vi "ConvStringIntoDouble (SubVI).vi"(1 "String In":string) -> (0 "Array Out":dbl[](array[numeric]))   [LabVIEW 2018]
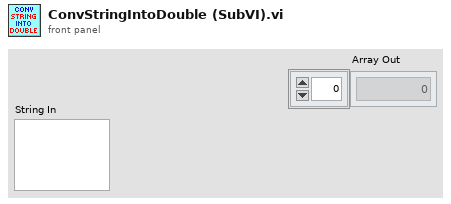
[diagram p1: front panel]
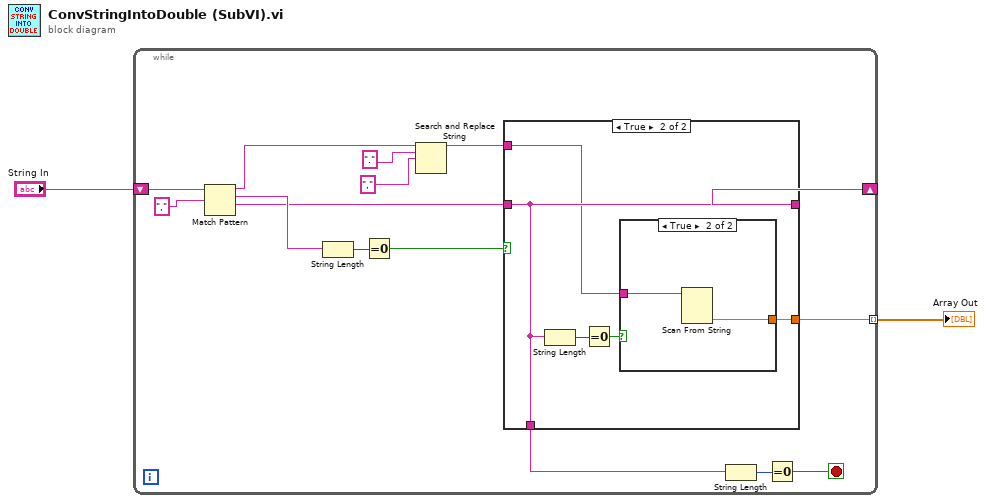
[diagram p0: block diagram]
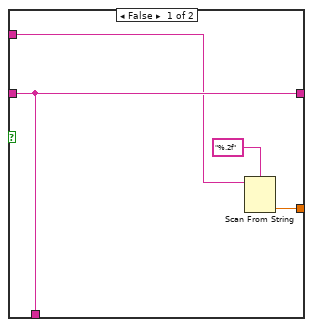
[diagram p2: hidden frame]
diagram:
  n1 = while {
    shift-right: [w13] -> _
    shift-left: "String In" -> [w17]
    tunnel: [w9] -> w2 mode=indexing
    stop <- w8 stop-if-true
    n2 = Match Pattern(string=w17, regular expression="," ("string")) -> (before substring=w3:string, match substring=w15:string, after substring=w12:string)  [unwired: 1 in, 1 out]
    n3 = String Length(string=w15) -> (length=w16:i32)
    n4 = Equal To 0?(x=w16) -> (x = 0?=w14:bool)
    n5 = Search and Replace String(input string=w3, search string=".", replace string="," ("replace string (\"\")")) -> (result string=w4:string)  [unwired: 5 in, 3 out]
    n6 = case shown="True" w14 {
      tunnel: [w19 w23] -> w13
      tunnel: w12 -> [w19 w23]
      tunnel: [w19 w23] -> w11
      tunnel: [w20 w24] -> w9
      tunnel: w4 -> [w18 w22]
      frame False {
        n7 = Scan From String(format string="%.2f", input string=w18) -> (output 1=w20:dbl)  [unwired: 3 in, 3 out]
      }
      frame True {
        n8 = String Length(string=w23) -> (length=w25:i32)
        n9 = Equal To 0?(x=w25) -> (x = 0?=w26:bool)
        n10 = case shown="True" w26 {
          tunnel: [_ w28] -> w24
          tunnel: w22 -> [_ w27]
          frame False {
          }
          frame True {
            n11 = Scan From String(input string=w27) -> (output 1=w28:dbl)  [unwired: 4 in, 3 out]
          }
        }
      }
    }
    n12 = String Length(string=w11) -> (length=w10:i32)
    n13 = Equal To 0?(x=w10) -> (x = 0?=w8:bool)
  }
  "Array Out" <- w2
